vi "Get Alias Mappings.vi"(8 "error in":errorcluster, 11 "endpoint aliases in":T3 format="%.0x") -> (0 "error out":errorcluster, 2 "alias mappings":T1[](array[typedef]), 3 "endpoint aliases out":T3 format="%.0x")   [LabVIEW 2020, in "Routing and Faulting Scripting.lvlib"]
doc: "Returns all alias names and mapped endpoints for the custom device."
uses:
  Routing and Faulting Scripting.lvlib
  <vilib>/NI VeriStand/Custom Device API/Custom Device Item Ref.ctl
  Shared/Alias Mapping.ctl
  Shared/Alias Endpoint.ctl
  <vilib>/NI VeriStand/Custom Device API/Custom Device API.lvlib
  Shared/Routing and Faulting Shared.lvlib
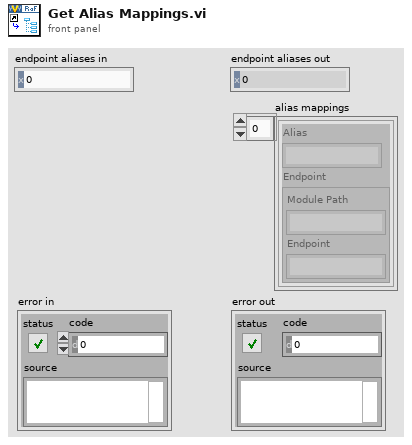
[diagram p1: front panel]
types:
  T1 = typedef "Routing and Faulting Shared.lvlib/Alias Mapping.ctl" = cluster{"Alias":string, "Endpoint":T2}
  T2 = typedef "Routing and Faulting Shared.lvlib/Alias Endpoint.ctl" = cluster{"Module Path":string, "Endpoint":string}
  T3 = typedef "Custom Device API.lvlib/Custom Device Item Ref.ctl" = u64
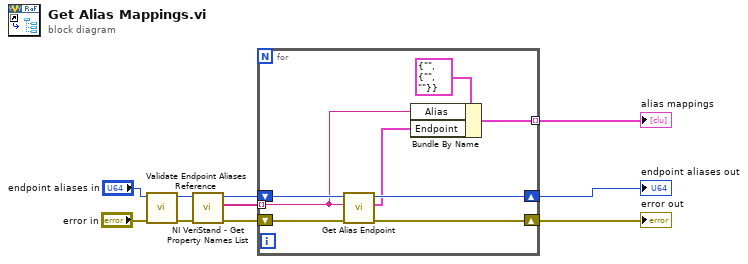
[diagram p0: block diagram]
diagram:
  n1 = call "Validate Endpoint Aliases Reference.vi"("error in"="error in", "endpoint aliases in"="endpoint aliases in") -> ("error out"=w3:errorcluster, "endpoint aliases out"=w1:T3)  [unwired: 8 in]
  n2 = call <vilib>:"NI VeriStand - Get Property Names List.vi"("error in (no error)"=w3, "Item Ref in"=w1) -> ("error out"=w9:errorcluster, "Property Names"=w10:string[], "Item Ref out"=w6:T3)  [unwired: 7 in]
  n3 = for {
    tunnel: w10 -> [w14] mode=indexing
    shift-right: [w11] -> w7
    shift-left: w9 -> [w16]
    tunnel: [w12] -> w4 mode=indexing
    shift-right: [w17] -> w5
    shift-left: w6 -> [w18]
    n4 = call "Get Alias Endpoint.vi"("error in"=w16, "alias"=w14, "endpoint aliases in"=w18) -> ("error out"=w11:errorcluster, "endpoint"=w13:T2, "endpoint aliases out"=w17:T3)  [unwired: 6 in]
    n5 = Bundle By Name(cluster=T1 {"Alias"="", "Endpoint"={"Module Path"="", "Endpoint"=""}} ("Alias Mapping"), "Alias"=w14, "Endpoint"=w13) -> (w12:T1)
  }
  "error out" <- w7
  "endpoint aliases out" <- w5
  "alias mappings" <- w4
